vi "Get Config.vi"(8 "error in (no error)":errorcluster) -> (0 "error out":errorcluster, 1 "Config ID":u32, 2 "Acustic Emision Frequency":i32, 3 "Photo Period":u32)   [LabVIEW 2023]
uses:
  <vilib>/httpClient/LabVIEWHTTPClient.lvlib
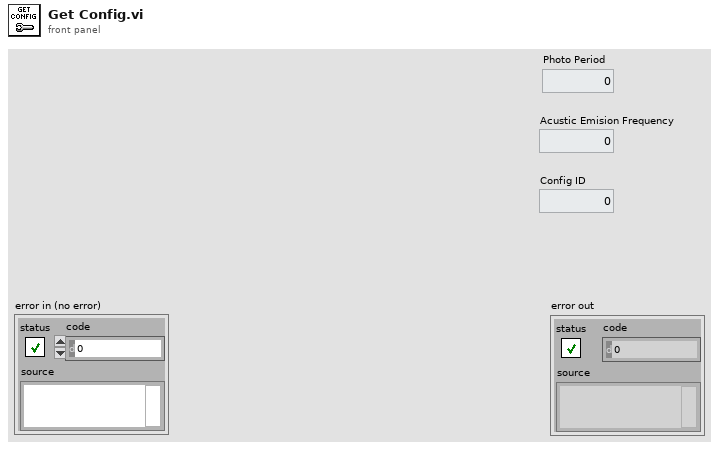
[diagram p1: front panel]
types:
  T1 = cluster{"id":i32, "interval":i32, "frequency":i32, "rgb_camera":bool, "hsi_camera":bool, "created_at":string}[]
  T2 = typedef "LabVIEWHTTPClient.lvlib/ClientHandle.ctl" = refnum<k1>
  T3 = cluster{"id":i32, "interval":i32, "frequency":i32, "rgb_camera":bool, "hsi_camera":bool, "created_at":string}
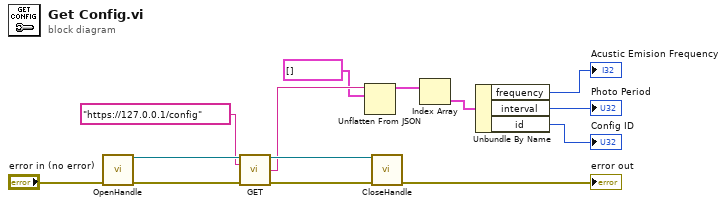
[diagram p0: block diagram]
diagram:
  n1 = call <vilib>:"OpenHandle.vi"("error in (no error)"="error in (no error)") -> ("client handle out"=w14:T2, "error out"=w10:errorcluster)  [unwired: 13 in]
  n2 = call <vilib>:"GET.vi"("client handle"=w14, "url"="https://127.0.0.1/config", "error in (no error)"=w10) -> ("client handle out"=w12:T2, "body"=w7:string, "error out"=w11:errorcluster)  [unwired: 9 in, 1 out]
  n3 = Unflatten From JSON(JSON string=w7, type and defaults=T1 []) -> (value=w4:T1)  [unwired: 5 in, 1 out]
  n4 = call <vilib>:"CloseHandle.vi"("client handle"=w12, "error in (no error)"=w11) -> ("error out"=→"error out":errorcluster)  [unwired: 13 in]
  n5 = Index Array(array=w4) -> (element=w3:T3)  [unwired: 1 in]
  n6 = Unbundle By Name(w3) -> ("frequency"=→"Acustic Emision Frequency":i32, "interval"=→"Photo Period":i32, "id"=→"Config ID":i32)
